vi "Init Plugin.vi"(8 "error in (no error)":errorcluster, 11 "PluginWithDatabase in":refnum<class "PluginWithDatabase.lvclass">) -> (0 "error out":errorcluster, 3 "PluginWithDatabase out":refnum<class "PluginWithDatabase.lvclass">)   [LabVIEW 2015, in "ActorManagement.lvlib" / "PluginWithDatabase.lvclass"]
uses:
  PluginWithDatabase.lvclass
  Plugin/Plugin.lvclass/Plugin.ctl
  PluginWithDatabase.lvclass/PluginWithDatabase.ctl
  DatabaseManagement/Database.lvclass
  UserManagement/Model/Model.lvclass
  Plugin/Plugin.lvclass
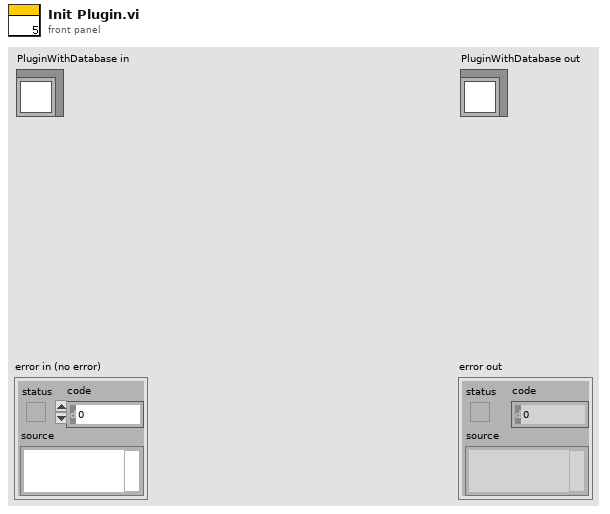
[diagram p1: front panel]
types:
  T1 = typedef "NI_Database_API.lvlib/DB Tools Column Info.ctl" = cluster{"column name":string, "data type":T2, "size":i32, "allow null?":bool}
  T2 = typedef "NI_Database_API.lvlib/DB Tools DataTypes.ctl" = enum16{"String", "Long (I32)", "Single (SGL)", "Double (DBL)", "Date/Time", "Binary"}
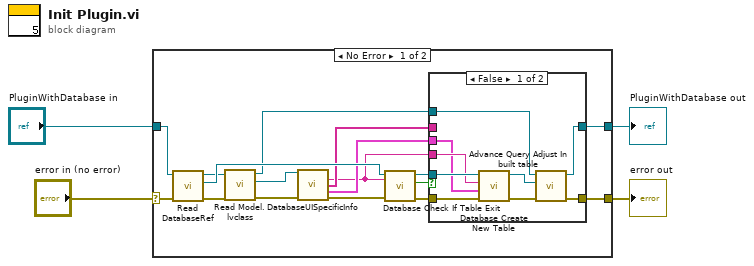
[diagram p0: block diagram]
diagram:
  n1 = case shown="No Error" "error in (no error)" {
    selector: "error in (no error)" -> [w16 w33]
    tunnel: "PluginWithDatabase in" -> [w14 w34]
    tunnel: [w15 w34] -> w2
    tunnel: [w18 w33] -> w1
    frame No Error {
      n2 = call "Read DatabaseRef.vi"("error in (no error)"=w16, "Plugin in"=w14) -> ("error out"=w12:errorcluster, "Database.lvlib:Database"=w17:refnum<class "Database.lvclass">, "Plugin out"=w13:refnum<class "PluginWithDatabase.lvclass">)  [unwired: 7 in]
      n3 = call "Read Model.lvclass.vi"("error in (no error)"=w12, "PluginWithDatabase in"=w13) -> ("error out"=w10:errorcluster, "UserManagement.lvlib:Model"=w11:refnum<class "Model.lvclass">, "PluginWithDatabase out"=w5:refnum<class "PluginWithDatabase.lvclass">)  [unwired: 7 in]
      n4 = call-dynamic "DatabaseUISpecificInfo.vi"("Model.lvclass"=w11, "error in (no error)"=w10) -> ("TableName"=w6:string, "TableItems"=w8:string[], "TableItemInfo"=w7:T1[], "error out"=w9:errorcluster)  [unwired: 9 in, 1 out]
      n5 = call "Database Check If Table Exit.vi"("error in (no error)"=w9, "Table"=w6, "Database in"=w17) -> ("error out"=w19:errorcluster, "Exit?"=w21:bool, "Database out"=w20:refnum<class "Database.lvclass">)  [unwired: 6 in]
      n6 = case shown="False" w21 {
        tunnel: w20 -> [w30 _]
        tunnel: w19 -> [w29 w32]
        tunnel: [w26 w32] -> w18
        tunnel: [w25 w31] -> w15
        tunnel: w8 -> [_ _]
        tunnel: w7 -> [w23 _]
        tunnel: w6 -> [w24 _]
        tunnel: w5 -> [w22 w31]
        frame False {
          n7 = call "Database Create New Table.vi"("error in (no error)"=w29, "column information"=w23, "table"=w24, "Database in"=w30) -> ("error out"=w27:errorcluster, "Database out"=w28:refnum<class "Database.lvclass">)  [unwired: 6 in]
          n8 = call-dynamic "Advance Query Adjust In built table.vi"("error in (no error)"=w27, "Database in"=w28, "PluginWithDatabase"=w22) -> ("error out"=w26:errorcluster, "PluginWithDatabase out"=w25:refnum<class "PluginWithDatabase.lvclass">)  [unwired: 7 in]
        }
        frame True {
        }
      }
    }
    frame Error {
    }
  }
  "error out" <- w1
  "PluginWithDatabase out" <- w2
